vi "GdsLanguage_ChecksumControl.vi"(8 "error in":errorcluster, 10 "ChesumControl":T1, 11 "LanguangeFileIn":path) -> (0 "error out":errorcluster, 3 "LanguangeFileOut":path)   [LabVIEW 2014]
uses:
  <resource>/Framework/Providers/Open_GDS/ClassProviders/Common/GdsLanguage/private/GdsLanguage_ChecksumCheckType.ctl
  <resource>/Framework/Providers/Open_GDS/SubVIs/GOOP_ErrorCodes.ctl
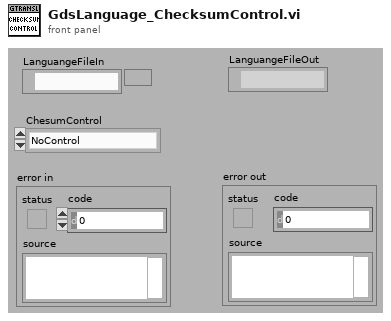
[diagram p1: front panel]
types:
  T1 = typedef "GdsLanguage_ChecksumCheckType.ctl" = enum16{"NoControl", "CheckChecksum", "AddChecksum"}
  T2 = typedef "GOOP_ErrorCodes.ctl" = enum16{"LicenseFileMissing", "LicenseFileNotCorrect", "NoProductAccessGranted", "AgreementNoAccepted", "NoValidProviderFound", "LicenseExpired", "LanguageUndefined", "LanguageFileMissing", "LanguageFileChecksumError", "DublicateLanguageTranslation", "LanguageStringIDNotFound", "CommunityLimitReached", "ClassFileLocked", "ClassFileReadOnly", "ProjectNotValid"}
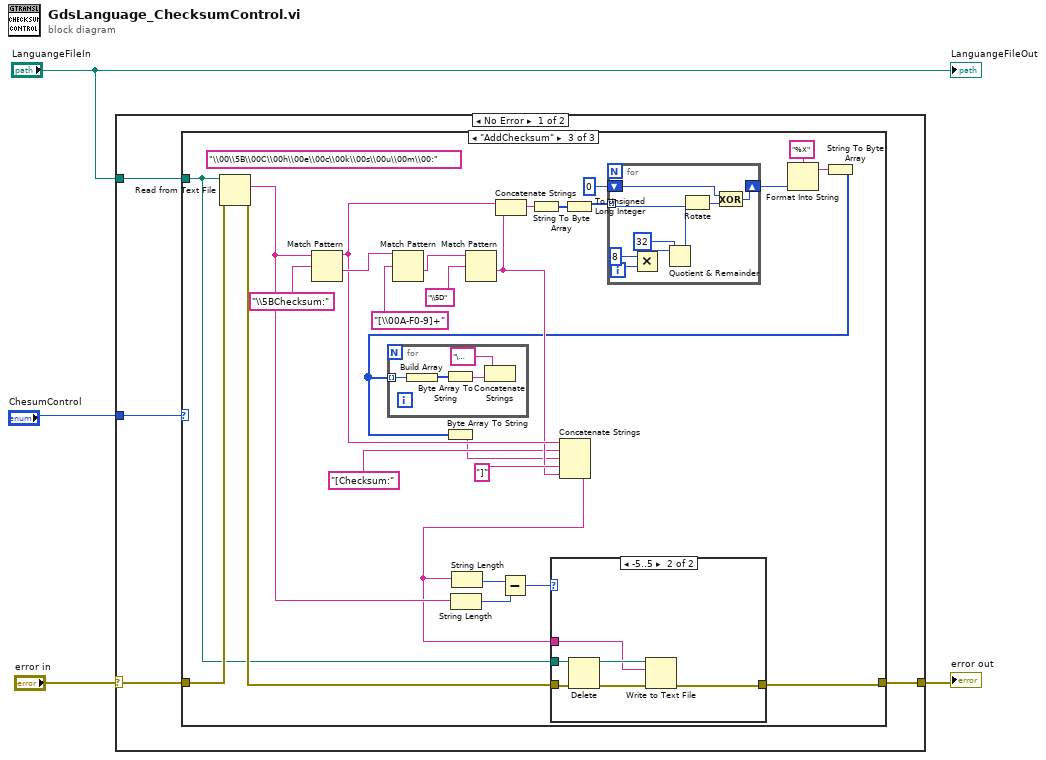
[diagram p0: block diagram]
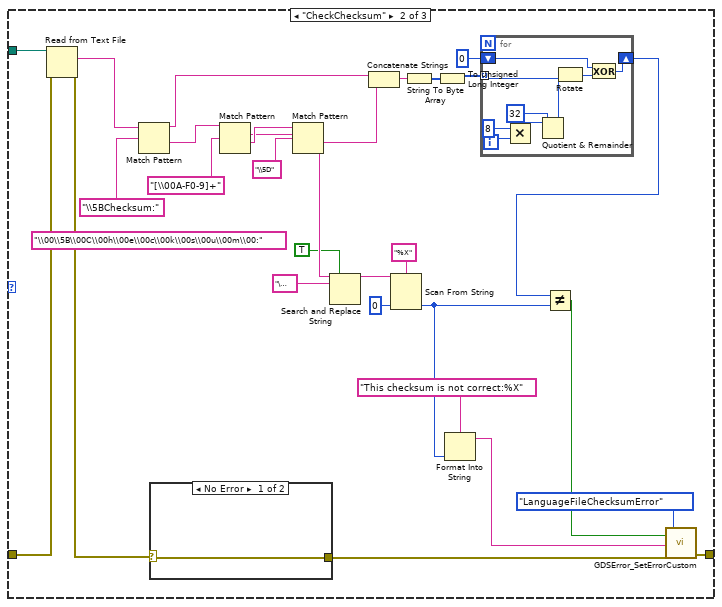
[diagram p3: hidden frame]
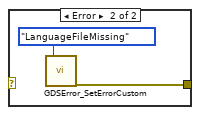
[diagram p4: hidden frame]
diagram:
  n1 = case shown="No Error" "error in" {
    selector: "error in" -> [w6 w98]
    tunnel: [w7 w98] -> w3
    tunnel: "LanguangeFileIn" -> [w5 _]
    tunnel: "ChesumControl" -> [w8 _]
    frame No Error {
      n2 = case shown="\"AddChecksum\"" w8 {
        tunnel: [w9 w22 w63] -> w7
        tunnel: w6 -> [w9 w37 w77]
        tunnel: w5 -> [_ w38 w56]
        frame "NoControl", Default {
        }
        frame "CheckChecksum" {
          (unwired) "\\00\\5B\\00C\\00h\\00e\\00c\\00k\\00s\\00u\\00m\\00:" ("regular expression")
          n3 = Read from Text File(file (use dialog)=w38, error in=w37) -> (text=w36:string, error out=w12:errorcluster)  [unwired: 2 in, 2 out]
          n4 = Match Pattern(string=w36, regular expression="\\5BChecksum:") -> (before substring=w31:string, after substring=w35:string)  [unwired: 1 in, 2 out]
          n5 = case shown="No Error" w12 {
            selector: w12 -> [w39 _]
            tunnel: [w39 w40] -> w11
            frame No Error {
            }
            frame Error {
              n6 = call <resource>:"GDSError_SetErrorCustom.vi"("UserDefinedCodes(+5000)"=GOOP_ErrorCodes."LanguageFileMissing") -> ("error out"=w40:errorcluster)  [unwired: 18 in]
            }
          }
          n7 = Match Pattern(string=w35, regular expression="[\\00A-F0-9]+") -> (match substring=w17:string, after substring=w33:string)  [unwired: 1 in, 2 out]
          n8 = Match Pattern(string=w33, regular expression="\\5D") -> (after substring=w30:string)  [unwired: 1 in, 3 out]
          n9 = Search and Replace String(replace all?=TRUE ("replace all? (F)"), input string=w17, search string="\u0000") -> (result string=w16:string)  [unwired: 5 in, 3 out]
          n10 = Concatenate Strings(w31, w30) -> (w26:string)
          n11 = Scan From String(format string="%X", input string=w16, default 1=u32 0 ("default value 1")) -> (output 1=w18:u32)  [unwired: 2 in, 3 out]
          n12 = String To Byte Array(string=w26) -> (unsigned byte array=w25:u8[])
          n13 = To Unsigned Long Integer(number=w25) -> (unsigned 32bit integer=w28:u32[])
          n14 = Format Into String(format string="This checksum is not correct:%X", w18) -> (resulting string=w19:string)  [unwired: 2 in, 1 out]
          n15 = for {
            tunnel: w28 -> [w50] mode=indexing
            shift-right: [w42] -> w24
            shift-left: u32 0 ("x") -> [w43]
            i -> [w49]
            n16 = Multiply(x=u32 8, y=w49) -> (x*y=w47:u32)
            n17 = Quotient & Remainder(x=w47, y=u32 32) -> (x-y*floor(x/y)=w45:u32)  [unwired: 1 out]
            n18 = Rotate(1:w50, 2:w45) -> (0:w44:u32)
            n19 = Exclusive Or(1:w44, 2:w43) -> (0:w42:u32)
          }
          n20 = Not Equal?(x=w24, y=w18) -> (x != y?=w21:bool)
          n21 = call <resource>:"GDSError_SetErrorCustom.vi"("status"=w21, "source"=w19, "error in (no error)"=w11, "UserDefinedCodes(+5000)"=GOOP_ErrorCodes."LanguageFileChecksumError") -> ("error out"=w22:errorcluster)  [unwired: 15 in]
        }
        frame "AddChecksum" {
          (unwired) "\\00\\5B\\00C\\00h\\00e\\00c\\00k\\00s\\00u\\00m\\00:" ("regular expression")
          n22 = Read from Text File(file (use dialog)=w56, error in=w77) -> (text=w68:string, error out=w64:errorcluster)  [unwired: 2 in, 2 out]
          n23 = Match Pattern(string=w68, regular expression="\\5BChecksum:") -> (before substring=w62:string, after substring=w76:string)  [unwired: 1 in, 2 out]
          n24 = Match Pattern(string=w76, regular expression="[\\00A-F0-9]+") -> (after substring=w74:string)  [unwired: 1 in, 3 out]
          n25 = String Length(string=w68) -> (length=w66:i32)
          n26 = Match Pattern(string=w74, regular expression="\\5D") -> (after substring=w57:string)  [unwired: 1 in, 3 out]
          n27 = Concatenate Strings(w62, w57) -> (w70:string)
          n28 = String To Byte Array(string=w70) -> (unsigned byte array=w69:u8[])
          n29 = To Unsigned Long Integer(number=w69) -> (unsigned 32bit integer=w72:u32[])
          n30 = for {
            tunnel: w72 -> [w97] mode=indexing
            shift-right: [w89] -> w61
            shift-left: u32 0 ("x") -> [w90]
            i -> [w96]
            n31 = Multiply(x=u32 8, y=w96) -> (x*y=w94:u32)
            n32 = Quotient & Remainder(x=w94, y=u32 32) -> (x-y*floor(x/y)=w92:u32)  [unwired: 1 out]
            n33 = Rotate(1:w97, 2:w92) -> (0:w91:u32)
            n34 = Exclusive Or(1:w91, 2:w90) -> (0:w89:u32)
          }
          n35 = Format Into String(format string="%X", w61) -> (resulting string=w59:string)  [unwired: 2 in, 1 out]
          n36 = String To Byte Array(string=w59) -> (unsigned byte array=w51:u8[])
          n37 = for {
            tunnel: w51 -> [w81] mode=indexing
            n38 = Build Array(w81) -> (w80:u8[])
            n39 = Byte Array To String(unsigned byte array=w80) -> (string=w79:string)
            n40 = Concatenate Strings("\u0000" ("string"), w79) -> ()  [unwired: 1 out]
          }
          n41 = Byte Array To String(unsigned byte array=w51) -> (string=w52:string)
          n42 = Concatenate Strings(w62, "[Checksum:" ("regular expression"), w52, "]" ("regular expression"), w57) -> (w55:string)
          n43 = String Length(string=w55) -> (length=w67:i32)
          n44 = Subtract(x=w67, y=w66) -> (x-y=w65:i32)
          n45 = case shown="-5..5" w65 {
            tunnel: w64 -> [w82 w88]
            tunnel: [w82 w84] -> w63
            tunnel: w56 -> [_ w87]
            tunnel: w55 -> [_ w83]
            frame Default {
            }
            frame -5..5 {
              n46 = Delete(path (use dialog)=w87, error in=w88) -> (deleted path=w85:path, error out=w86:errorcluster)  [unwired: 3 in, 1 out]
              n47 = Write to Text File(file (use dialog)=w85, text=w83, error in=w86) -> (error out=w84:errorcluster)  [unwired: 1 in, 2 out]
            }
          }
        }
      }
    }
    frame Error {
    }
  }
  "error out" <- w3
  "LanguangeFileOut" <- "LanguangeFileIn"
